vi "Set Multi-Line Package Attribute Value.vi"(0 "package attributes string in":string, 5 "package attribute name":string, 7 "synopsis":string, 9 "description":string, 11 "error in (no error)":errorcluster, 12 "add nonexisting attribute to string (T)":bool=TRUE) -> (4 "package attributes string out":string, 6 "new attribute added to string?":bool, 8 "attribute found?":bool, 15 "error out":errorcluster)   [LabVIEW 2014, in "NIPM_API.lvlib"]
doc: "Sets the value for an attribute in a package attribute string.\n\npackage attributes string in - This is the initial string containing the package attributes. For example, this string could come from reading the contents of an unpacked package's control file.\n\npackage attribute name - This is the name of the attribute whose value you want to change.\n\npackage attribute value - This is the value you want to set the attribute to.\n\nadd nonexisting attribute to string - If this VI does not find the \"package attribute name\" in the \"package attributes string in\" string, this input determines whether this VI will add the \"package attribute name\" and \"package attribute value\" to the \"package attribute string\".\nNote: If this input is TRUE, but the \"package attribute value\" is a default value (\"\"), then this VI will not add a new attribute to the string.\n\nnew attribute added to string? - This output will be TRUE if a new attribute (did not exist in the incoming \"package attributes string in\" string) was added to the package attributes string.\n\nattribute found? - This output will be TRUE if the \"package attribute name\" was found in the incoming \"package attributes string in\" string."
uses:
  NIPM_API.lvlib
  <vilib>/Utility/error.llb/whitespace.ctl
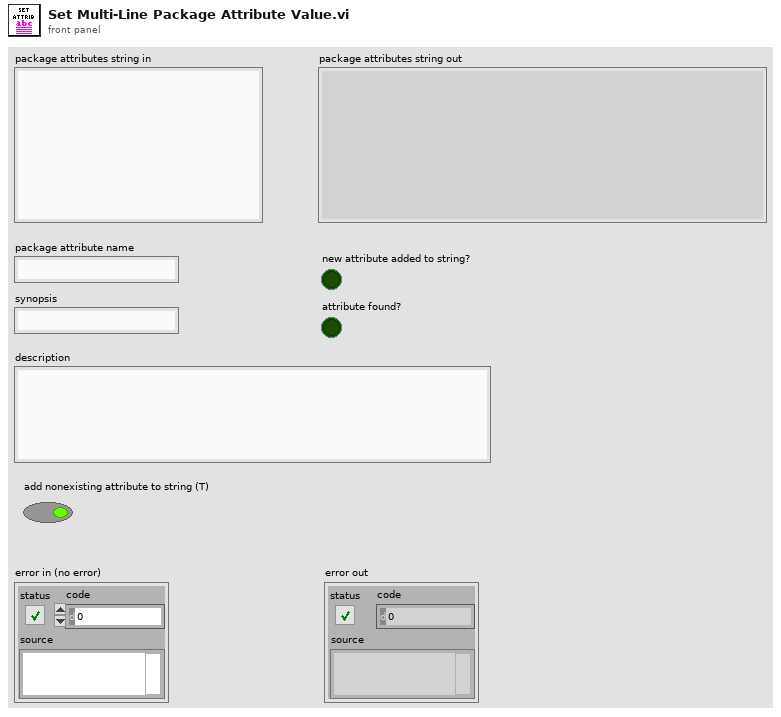
[diagram p1: front panel]
types:
  T1 = typedef "whitespace.ctl" = u16
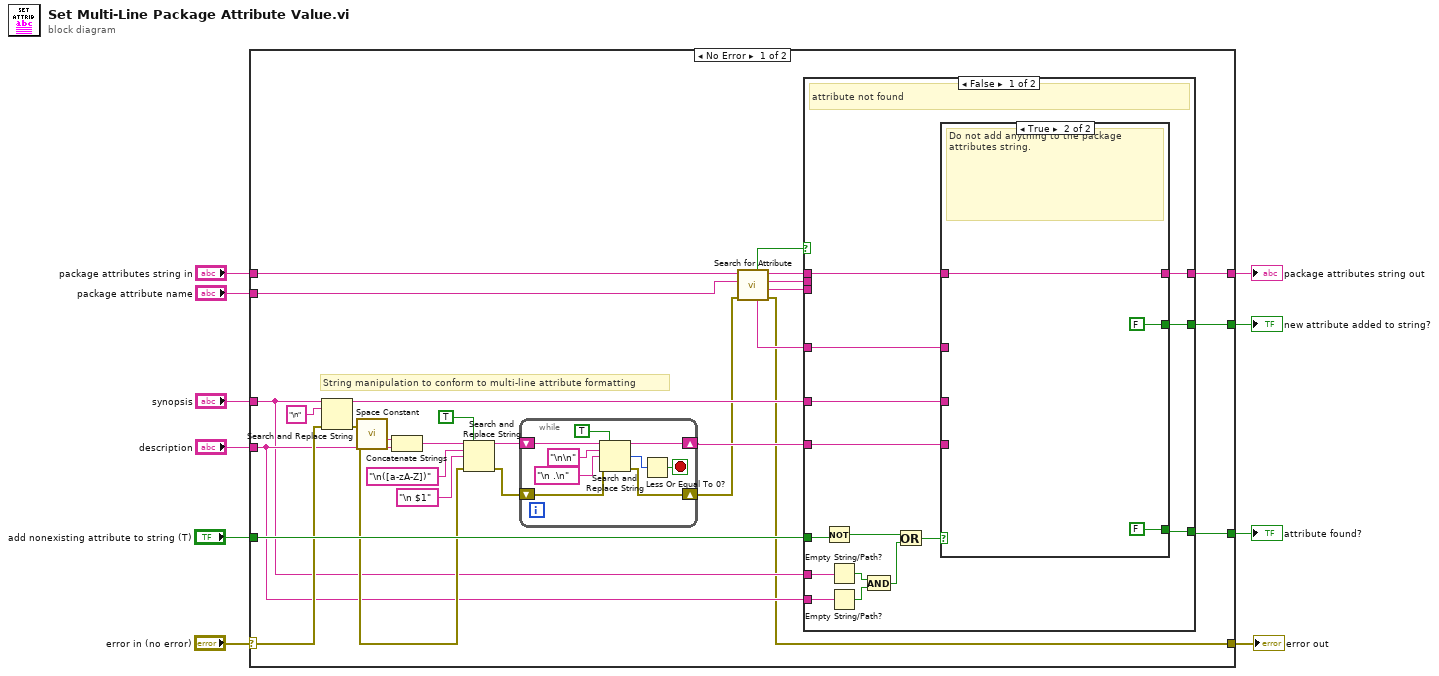
[diagram p0: block diagram]
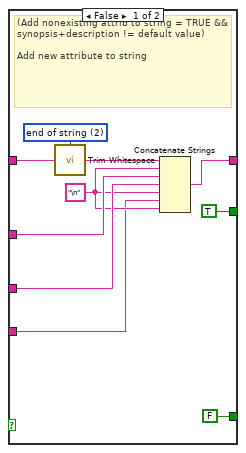
[diagram p2: hidden frame]
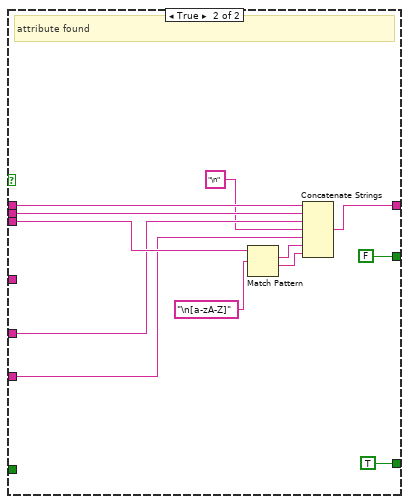
[diagram p3: hidden frame]
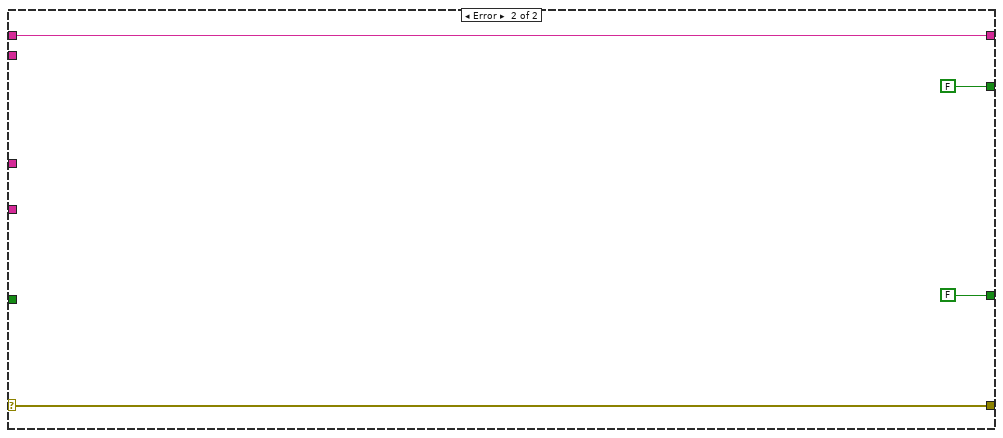
[diagram p4: hidden frame]
diagram:
  n1 = case shown="No Error" "error in (no error)" {
    selector: "error in (no error)" -> [w31 w90]
    tunnel: [w37 w87] -> w10
    tunnel: "package attribute name" -> [w13 _]
    tunnel: "package attributes string in" -> [w19 w87]
    tunnel: [w11 w90] -> w6
    tunnel: "description" -> [w21 _]
    tunnel: [w36 FALSE] -> w4
    tunnel: "add nonexisting attribute to string (T)" -> [w35 _]
    tunnel: [w34 FALSE] -> w2
    tunnel: "synopsis" -> [w20 _]
    frame No Error {
      # "String manipulation to conform to multi-line attribute formatting"
      n2 = Search and Replace String(input string=w20, search string="\n" ("regular expression"), error in=w31) -> (result string=w32:string, error out=w23:errorcluster)  [unwired: 5 in, 2 out]
      n3 = call <vilib>:"Space Constant.vi"() -> ("String"=w30:string)
      n4 = Concatenate Strings(w30, w21) -> (w27:string)
      n5 = Search and Replace String(replace all?=TRUE ("replace all? (F)"), input string=w27, search string="\n([a-zA-Z])" ("Package Attribute Name"), replace string="\n $1" ("Package Attribute Name"), error in=w23) -> (result string=w28:string, error out=w24:errorcluster)  [unwired: 3 in, 2 out]
      n6 = while {
        shift-right: [w43] -> w29
        shift-left: w28 -> [w46]
        shift-right: [w39] -> w12
        shift-left: w24 -> [w40]
        stop <- w41 stop-if-true
        n7 = Search and Replace String(replace all?=TRUE ("replace all? (F)"), input string=w46, search string="\n\n" ("regular expression"), replace string="\n .\n" ("regular expression"), error in=w40) -> (result string=w43:string, number of replacements=w42:i32, error out=w39:errorcluster)  [unwired: 3 in, 1 out]
        n8 = Less Or Equal To 0?(x=w42) -> (x <= 0?=w41:bool)
      }
      n9 = call "Search for Attribute.vi"("error in (no error)"=w12, "package attribute name"=w13, "package attributes CLI string in"=w19) -> ("error out"=w11:errorcluster, "string after attribute"=w16:string, "string matching attribute"=w17:string, "string before attribute"=w18:string, "package attribute string"=w14:string, "attribute found?"=w15:bool)  [unwired: 3 in]
      n10 = case shown="False" w15 {
        tunnel: w18 -> [w61 w86]
        tunnel: w17 -> [_ w85]
        tunnel: w29 -> [w57 w77]
        tunnel: w16 -> [_ w84]
        tunnel: [w59 w83] -> w37
        tunnel: [w60 FALSE] -> w36
        tunnel: w14 -> [w58 _]
        tunnel: w35 -> [w54 _]
        tunnel: [w56 TRUE] -> w34
        tunnel: w32 -> [w55 w78]
        tunnel: w21 -> [w50 _]
        tunnel: w20 -> [w51 _]
        frame False {
          # "attribute not found"
          n11 = Not(x=w54) -> (.not. x?=w52:bool)
          n12 = Empty String/Path?(string/path=w51) -> (empty?=w49:bool)
          n13 = Empty String/Path?(string/path=w50) -> (empty?=w48:bool)
          n14 = And(x=w49, y=w48) -> (x .and. y?=w47:bool)
          n15 = Or(x=w52, y=w47) -> (x .or. y?=w53:bool)
          n16 = case shown="True" w53 {
            tunnel: w61 -> [w71 w74]
            tunnel: [TRUE FALSE] -> w60
            tunnel: [w69 w74] -> w59
            tunnel: w58 -> [w68 _]
            tunnel: w57 -> [w62 _]
            tunnel: [FALSE FALSE] -> w56
            tunnel: w55 -> [w64 _]
            frame False {
              w63 = "\n"
              w66 = T1 2 items=["both", "start of string", "end of string"] ("location (both)")
              # "(Add nonexisting attrib to string = TRUE && synopsis+description != default value)\n\nAdd new attribute to string"
              n17 = call <vilib>:"Trim Whitespace.vi"("string"=w71, "location (both)"=w66) -> ("trimmed string"=w67:string)
              n18 = Concatenate Strings(w67, w63, w68, w64, w63, w62, w63) -> (w69:string)
            }
            frame True {
              # "Do not add anything to the package attributes string."
            }
          }
        }
        frame True {
          # "attribute found"
          n19 = Match Pattern(string=w84, regular expression="\n[a-zA-Z]" ("Package Attribute Name")) -> (match substring=w81:string, after substring=w80:string)  [unwired: 1 in, 2 out]
          n20 = Concatenate Strings(w86, w85, w78, "\n" ("regular expression"), w77, w81, w80) -> (w83:string)
        }
      }
    }
    frame Error {
    }
  }
  "package attributes string out" <- w10
  "error out" <- w6
  "new attribute added to string?" <- w4
  "attribute found?" <- w2
